vi "Cyclic Prefix Removal.vi"(10 "sample timing in":T2, 11 "channels in":T1) -> (2 "sample timing out":T2, 3 "channels out":T1)   [LabVIEW 2020]
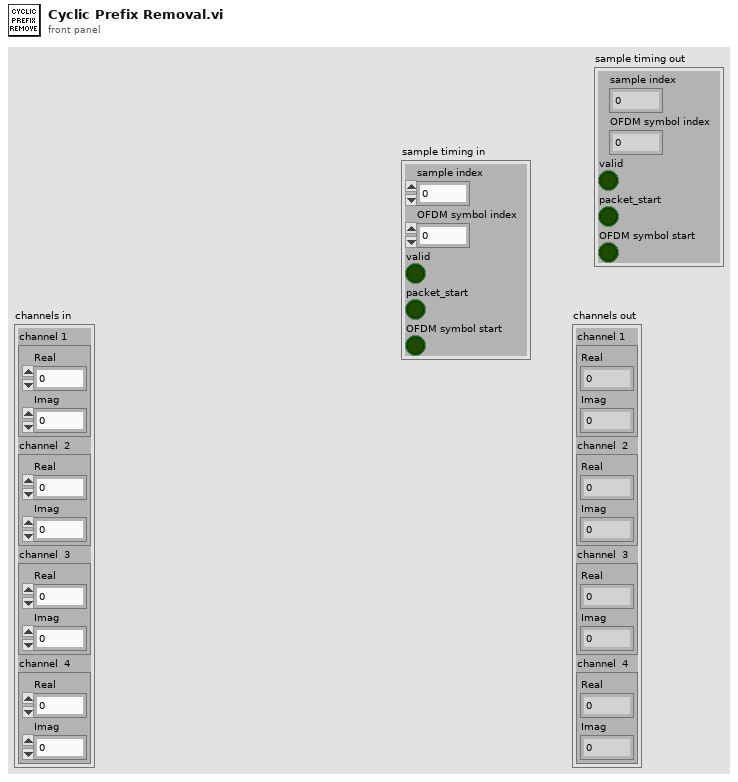
[diagram p1: front panel]
types:
  T1 = cluster{"channel 1 ":cluster{"Real":fxp<+/-,16,3>, "Imag":fxp<+/-,16,3>}, "channel  2":cluster{"Real":fxp<+/-,16,3>, "Imag":fxp<+/-,16,3>}, "channel  3":cluster{"Real":fxp<+/-,16,3>, "Imag":fxp<+/-,16,3>}, "channel  4":cluster{"Real":fxp<+/-,16,3>, "Imag":fxp<+/-,16,3>}}
  T2 = cluster{"sample index":u16, "OFDM symbol index":u16, "valid":bool, "packet_start":bool, "OFDM symbol start":bool}
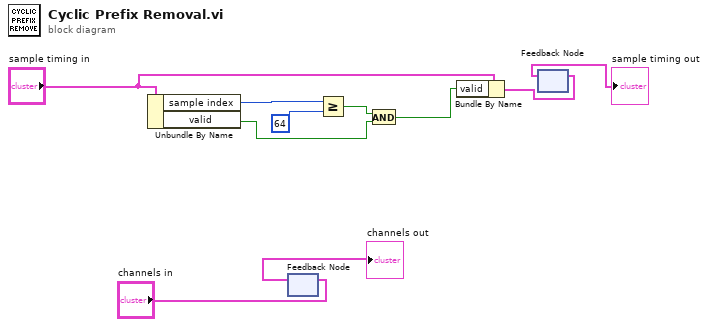
[diagram p0: block diagram]
diagram:
  n1 = Unbundle By Name("sample timing in") -> ("sample index"=w10:u16, "valid"=w7:bool)
  n2 = feedback #1() -> (→"channels out":T1)  [unwired: 1 in]
  n3 = feedback-in #1("channels in") -> ()
  n4 = Greater Or Equal?(x=w10, y=u16 64) -> (x >= y?=w8:bool)
  n5 = And(x=w8, y=w7) -> (x .and. y?=w5:bool)
  n6 = Bundle By Name(cluster="sample timing in", "valid"=w5) -> (w3:T2)
  n7 = feedback #2() -> (→"sample timing out":T2)  [unwired: 1 in]
  n8 = feedback-in #2(w3) -> ()
